vi "http_select_header_field.vi"(10 "Name":string, 11 "Request Header Fields":T1[](array[typedef])) -> (2 "found":bool, 3 "Header Field":T1)   [LabVIEW 2011]
uses:
  http_field.ctl
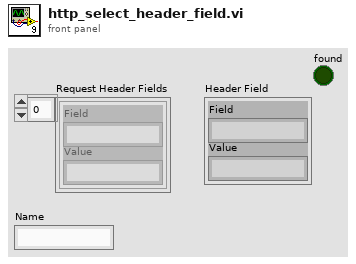
[diagram p1: front panel]
types:
  T1 = typedef "http_field.ctl" = cluster{"Field":string, "Value":string}
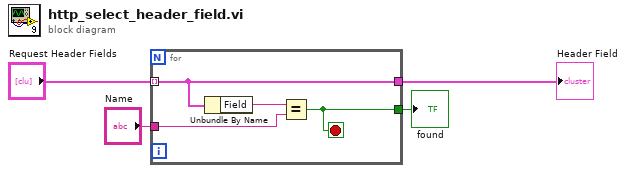
[diagram p0: block diagram]
diagram:
  n1 = for {
    tunnel: "Request Header Fields" -> [w5] mode=indexing
    tunnel: "Name" -> [w7]
    tunnel: [w6] -> w1
    tunnel: [w5] -> w4
    stop <- w6 stop-if-true
    n2 = Unbundle By Name(w5) -> ("Field"=w8:string)
    n3 = Equal?(x=w8, y=w7) -> (x = y?=w6:bool)
  }
  "Header Field" <- w4
  "found" <- w1
